vi "SerialPort.Connect.vi"(8 "error in (no error)":errorcluster, 11 "SerialPort in":refnum<class "SerialPort.lvclass">) -> (0 "error out":errorcluster, 2 "State":T1, 3 "SerialPort out":refnum<class "SerialPort.lvclass">)   [LabVIEW 2018, in "SerialPort.lvclass"]
uses:
  SerialPort.lvclass
  Controls/SerialPort.Status Enum.ctl
  SerialPort.lvclass/SerialPort.ctl
  Utils/Errors/Error.Error Code List.ctl
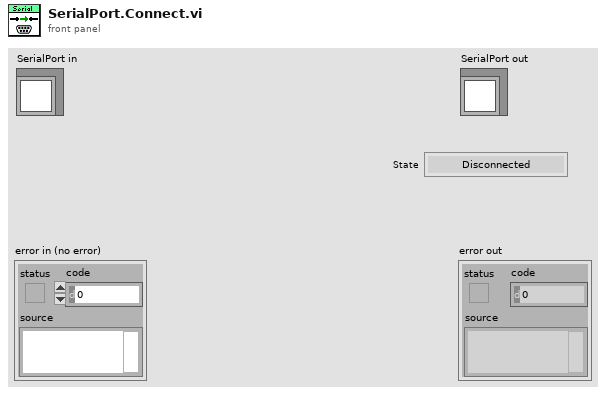
[diagram p1: front panel]
types:
  T1 = typedef "SerialPort.Status Enum.ctl" = enum16{"Disconnected", "Connecting", "Connected"}
  T2 = typedef "Error.Error Code List.ctl" = i32
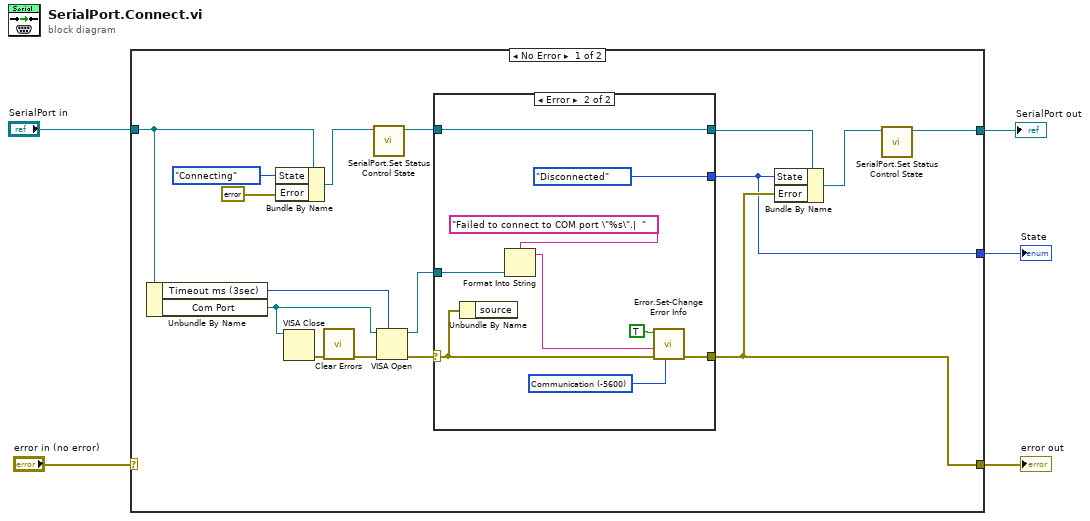
[diagram p0: block diagram]
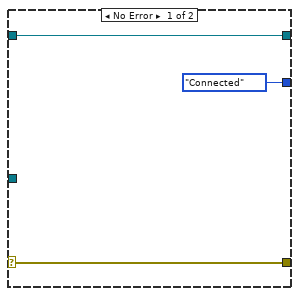
[diagram p2: hidden frame]
diagram:
  n1 = case shown="No Error" "error in (no error)" {
    selector: "error in (no error)" -> [_ w35]
    tunnel: [w18 w35] -> w4
    tunnel: [w19 w34] -> w2
    tunnel: "SerialPort in" -> [w13 w34]
    tunnel: [w10 _] -> w1
    frame No Error {
      n2 = Unbundle By Name(w13) -> ("Timeout ms (3sec)"=w21:u32, "Com Port"=w6:refnum<visa-resource-name>)
      n3 = Bundle By Name(cluster=w13, "State"=SerialPort.Status_Enum."Connecting", "Error"=errorcluster {"status"=FALSE, "code"=0, "source"=""}) -> (w11:refnum<class "SerialPort.lvclass">)
      n4 = VISA Close(VISA resource name=w6) -> (error out=w7:errorcluster)  [unwired: 1 in]
      n5 = call <vilib>:"Clear Errors.vi"("error in (no error)"=w7) -> ("error out"=w8:errorcluster)  [unwired: 5 in, 1 out]
      n6 = call "SerialPort.Set Status Control State.vi"("SerialPort in"=w11) -> ("SerialPort out"=w12:refnum<class "SerialPort.lvclass">)  [unwired: 9 in, 1 out]
      n7 = VISA Open(timeout (0)=w21, error in (no error)=w8, VISA resource name=w6) -> (VISA resource name=w9:refnum<visa-resource-name>, error out=w20:errorcluster)  [unwired: 2 in]
      n8 = case shown="Error" w20 {
        selector: w20 -> [w22 w27]
        tunnel: [w22 w26] -> w18
        tunnel: w12 -> [w23 w33]
        tunnel: [w23 w33] -> w17
        tunnel: [SerialPort.Status_Enum."Connected" ("State") SerialPort.Status_Enum."Disconnected" ("State")] -> w10
        tunnel: w9 -> [_ w30]
        frame No Error {
        }
        frame Error {
          w29 = T2 -5600 items=["No Error"=0, "Abort"=-2, "Misc"=-5000, "Fixture Error"=-5100, "File IO - General"=-5200, "FIle IO - Config Error"=-5201, "Instrument - General"=-5300, "Instrument - Serial Com"=-5301, "Instrument - Camera"=-5302, "Instrument - PS"=-5303, "Instrument - Oscilloscope"=-5304, "Instrument - Function Gen"=-5305, "Instrument - Load"=-5306, "Instrument - Meter"=-5307, "Instrument - Power Control"=-5308, "Instrument - Motion"=-5309, "Instrument - RF"=-5310, "System Exe"=-5400, "Image Processing"=-5500, "Communication"=-5600, "Script - Syntax Error"=-6000, "Script - Invalid Name or Param"=-6100, "Script - Timeout"=-6200, "Invalid Data"=-6300] ("Std Code")
          n9 = Unbundle By Name(w27) -> ()  [unwired: 1 out]
          n10 = Format Into String(format string="Failed to connect to COM port \"%s\".|  ", w30) -> (resulting string=w25:string)  [unwired: 2 in, 1 out]
          n11 = call "Error.Set-Change Error Info.vi"("Std Code"=w29, "error in"=w27, "Description"=w25, "Set Error"=TRUE) -> ("error out"=w26:errorcluster)  [unwired: 7 in]
        }
      }
      n12 = Bundle By Name(cluster=w17, "State"=w10, "Error"=w18) -> (w16:refnum<class "SerialPort.lvclass">)
      n13 = call "SerialPort.Set Status Control State.vi"("SerialPort in"=w16) -> ("SerialPort out"=w19:refnum<class "SerialPort.lvclass">)  [unwired: 9 in, 1 out]
    }
    frame Error {
    }
  }
  "error out" <- w4
  "SerialPort out" <- w2
  "State" <- w1
